vi "StringArrayToMultiLineString.vi"(10 "Reset":bool, 11 "String":string) -> (3 "MultiLineString":string)   [LabVIEW 2017]
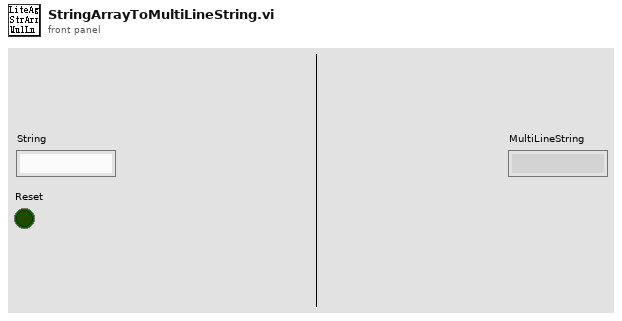
[diagram p1: front panel]
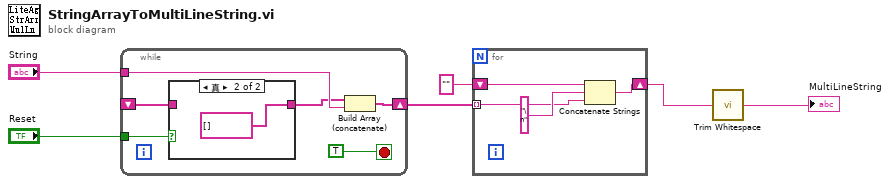
[diagram p0: block diagram]
diagram:
  n1 = while {
    tunnel: "String" -> [w12]
    shift-right: [w11] -> w2
    shift-left: _ -> [w8]
    tunnel: "Reset" -> [w9]
    stop <- TRUE stop-if-true
    n2 = case shown="真" w9 {
      tunnel: w8 -> [w13 _]
      tunnel: [w13 string[] []] -> w7
      frame False {
      }
      frame True {
      }
    }
    n3 = Build Array (concatenate)(w7, w12) -> (w11:string[])
  }
  n4 = for {
    tunnel: w2 -> [w15] mode=indexing
    shift-right: [w17] -> w6
    shift-left: "" -> [w16]
    n5 = Concatenate Strings(w16, "\n" ("字符串"), w15) -> (w17:string)
  }
  n6 = call <vilib>:"Trim Whitespace.vi"("string"=w6) -> ("trimmed string"=→"MultiLineString":string)  [unwired: 1 in]
